vi "_Main_LookOnly_V2.0_3el_5el.vi"() -> ()   [LabVIEW 2017]
uses:
  <vilib>/Instr/_visa.llb/VISA Configure Serial Port (Instr).vi
panel:
  in  "5electrodes":bool=TRUE
  out "Channel 4, V":dbl format="%#_5g"
  in  "DAC 1 LIMIT, V":dbl min=-50.0 max=50.0 format="%#_5g"
  in  "DAC 2, V":dbl min=-10.0 max=10.0 format="%#_5g"
  in  "DAC 1, V":dbl min=-50.0 max=50.0 format="%#_5g"
  out "DAC1volt, V":dbl
  out "Field LOG":cluster{dbl[], dbl[]}(graph)
  out "Bytes at Port":u32
  out "RecTry":i32
  out "Field, kV/cm":dbl
  out "VoltageRes, V":dbl
  out "PlotPoints":cluster{"Time":dbl[], "Voltage":dbl[]}(graph)={"Time"=[0.0, 0.00037111111108161925, 0.000510833333311085, 0.0006505555555405509, 0.0007766666666915019, 0.0009172222221968695, 0.0010569444444263353, 0.0011958333333152243, 0.0013350000000274223], "Voltage"=[5.89, 5.89, 5.89, 5.89, 5.89, 5.89, 5.89, 5.89, 5.89]}
  out "VoltageBelow, V":dbl
  out "Current, mA":dbl format="%#_4g"
  out "Channel 3, V":dbl format="%#_5g"
  out "Channel 2, V":dbl format="%#_5g"
  out "Channel 1, V":dbl format="%#_5g"
  in  "Stop Button":bool
  in  "Start Button":bool
  in  "film H, nm":dbl=50.0
  in  "COM port":refnum<visa-resource-name>
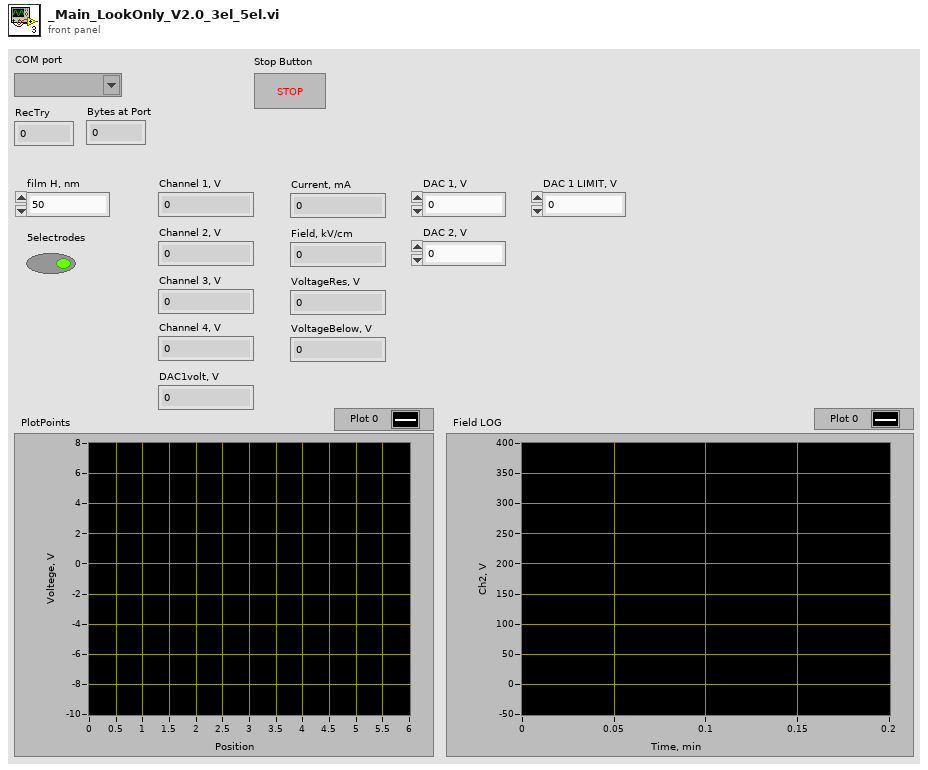
[diagram p1: front panel]
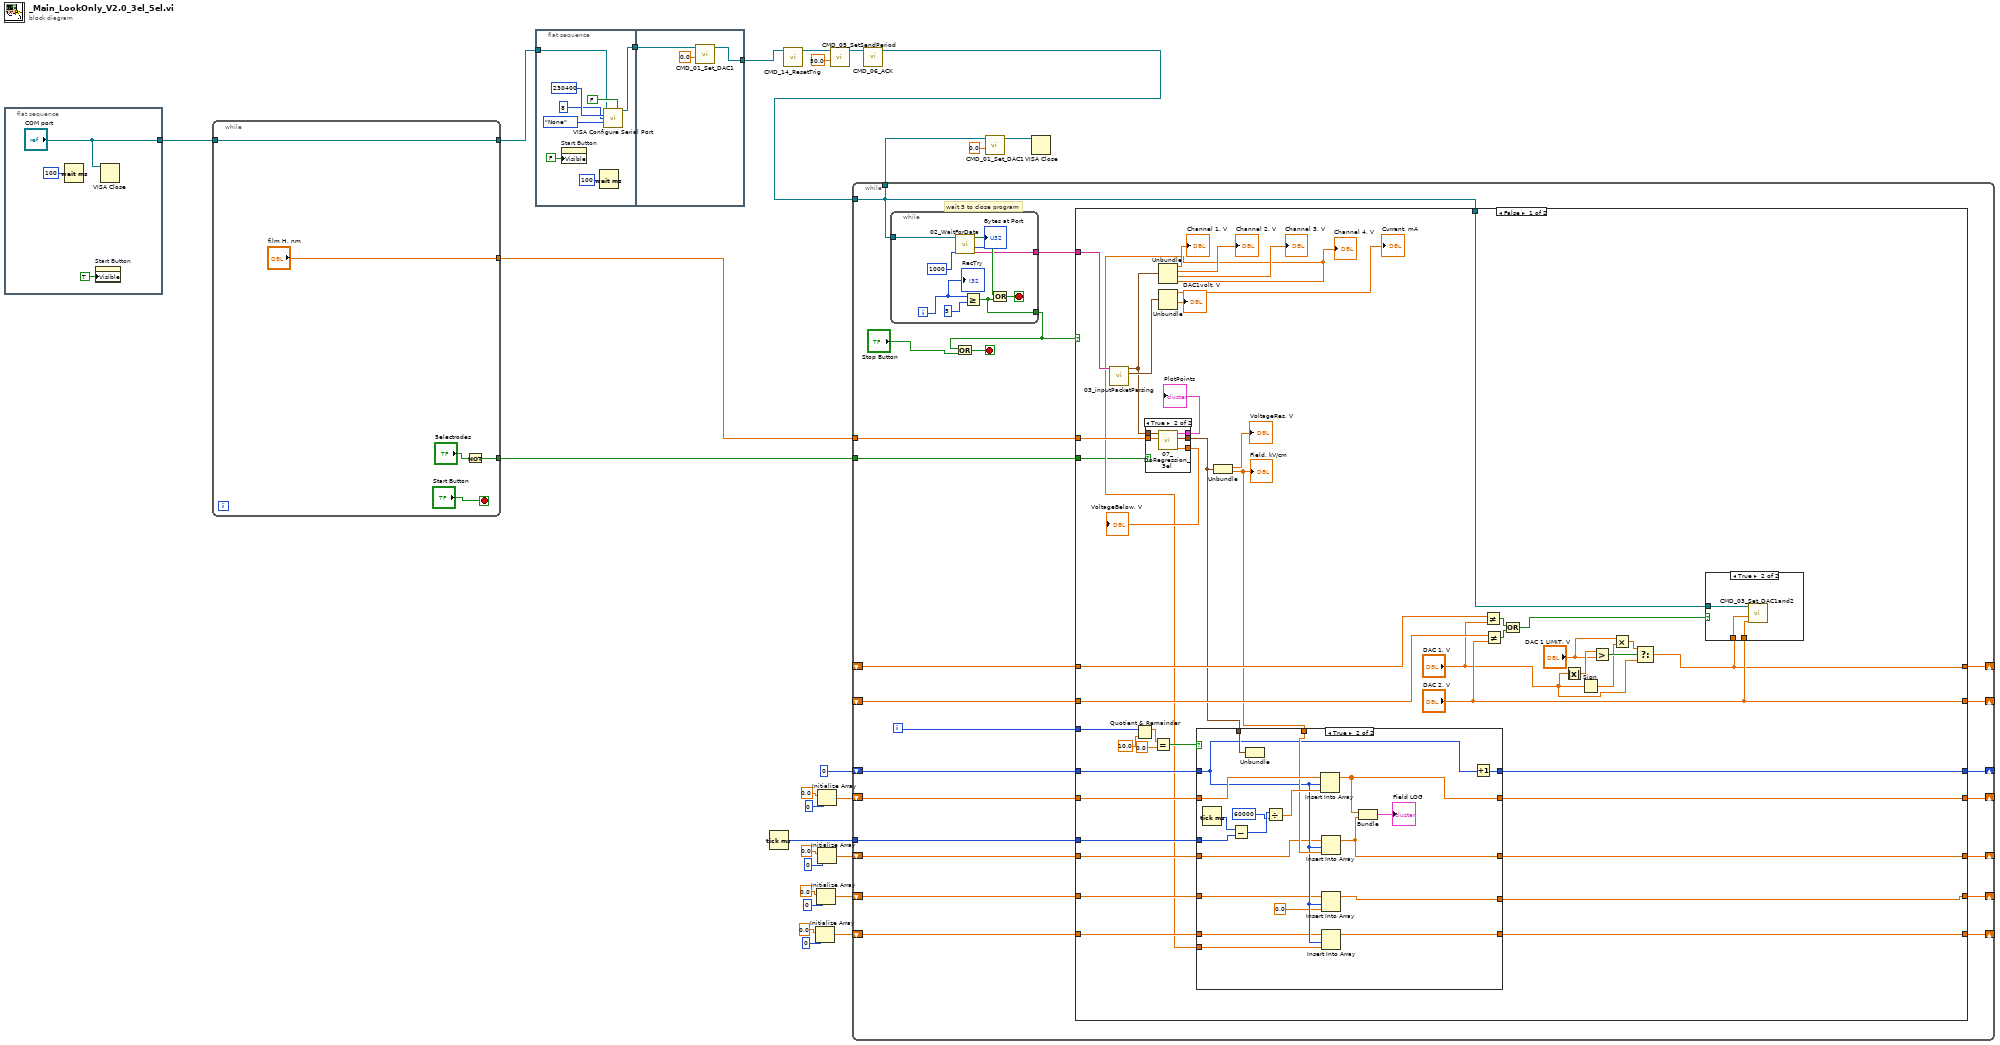
[diagram p0: block diagram]
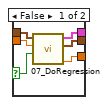
[diagram p2: hidden frame]
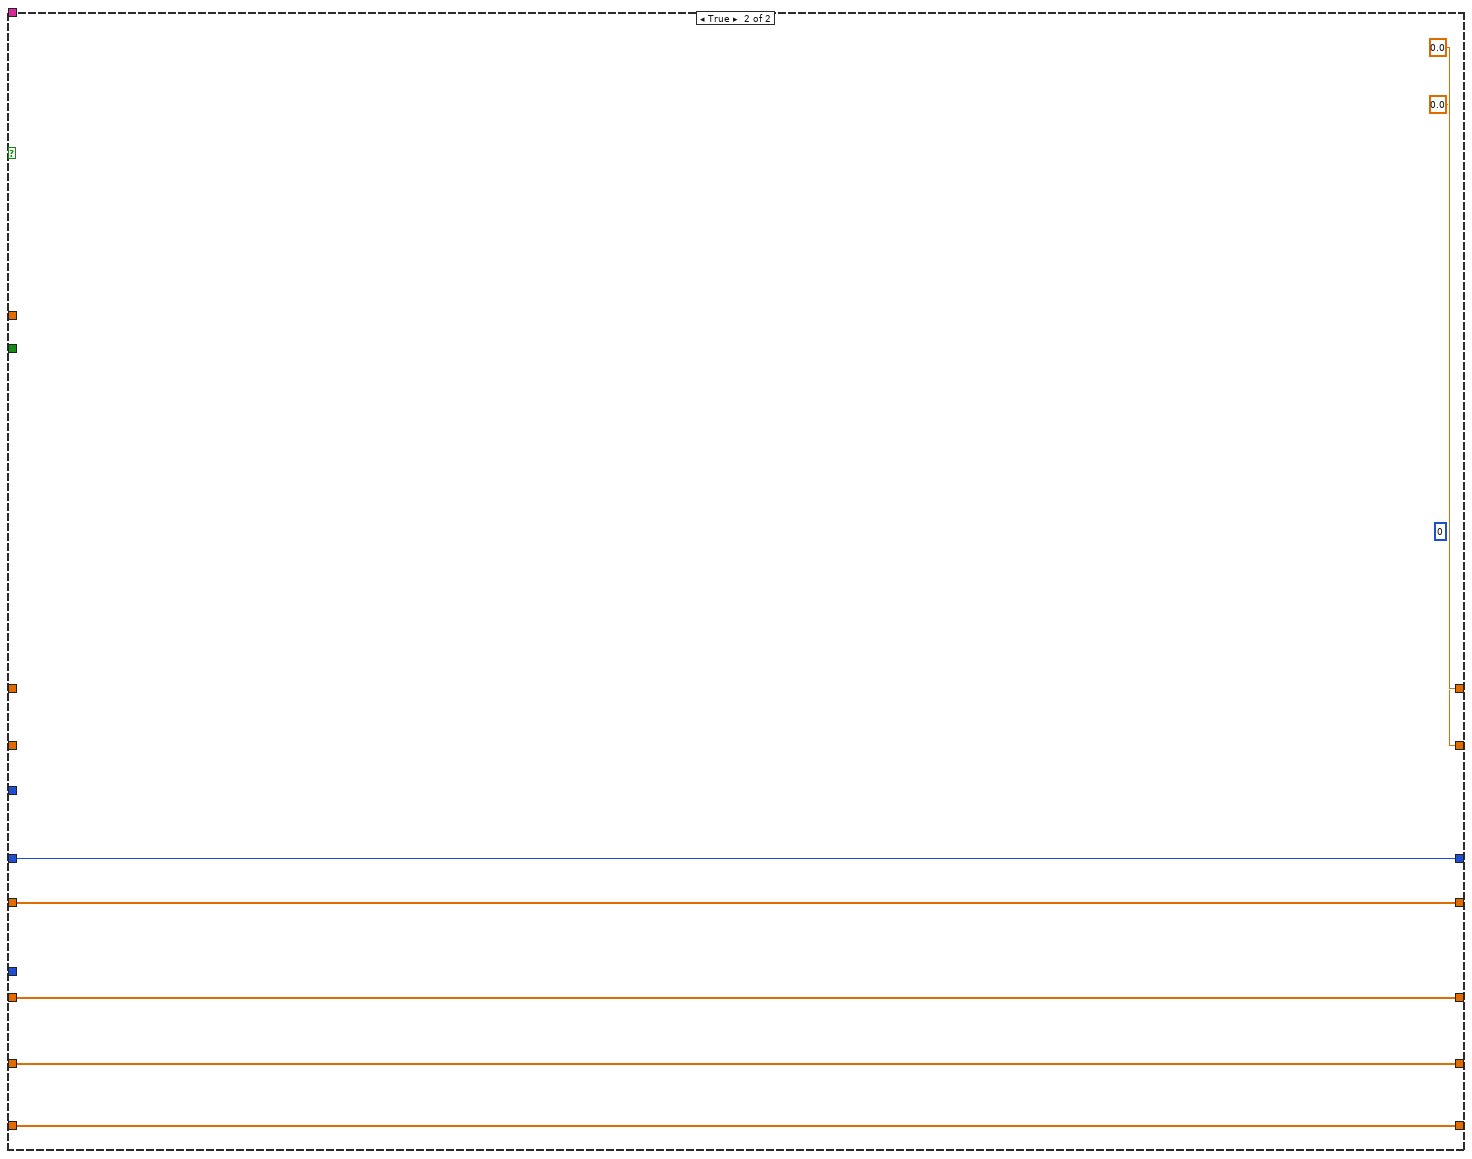
[diagram p5: hidden frame]
diagram:
  n1 = flat-sequence {
    tunnel: ["COM port"] -> w27
    frame #0 {
      n2 = Wait (ms)(milliseconds to wait=u32 100) -> ()  [unwired: 1 out]
      n3 = property on="Start Button" class="Bool"("Visible"=TRUE) -> ()  [unwired: 2 in, 2 out]
      n4 = VISA Close(VISA resource name="COM port") -> ()  [unwired: 1 in, 1 out]
    }
  }
  n5 = while {
    tunnel: w27 -> [w34]
    tunnel: [w34] -> w26
    tunnel: ["film H, nm"] -> w25
    tunnel: [w32] -> w1
    stop <- "Start Button" stop-if-true
    n6 = Not(x="5electrodes") -> (.not. x?=w32:bool)
  }
  n7 = flat-sequence {
    tunnel: w26 -> [w39]
    tunnel: [w38] -> w16
    tunnel: [w46] -> w23
    tunnel: w16 -> [w45]
    frame #0 {
      n8 = property on="Start Button" class="Bool"("Visible"=FALSE) -> ()  [unwired: 2 in, 2 out]
      n9 = Wait (ms)(milliseconds to wait=u32 100) -> ()  [unwired: 1 out]
      n10 = call-poly "VISA Configure Serial Port"("VISA resource name"=w39, "Enable Termination\nChar (T)"=FALSE ("Enable Termination\nChar (T)"), "baud rate (9600)"=u32 230400, "data bits (8)"=u16 8, "parity (0:none)"=enum16{"None", "Odd", "Even", "Mark", "Space"}."None") -> ("VISA resource name out"=w38:refnum<visa-resource-name>)  [unwired: 9 in, 1 out]
    }
    frame #1 {
      n11 = call "CMD_01_Set_DAC1.vi"("Input, V"=0.0, "VISA resource name"=w45) -> ("VISA resource name out"=w46:refnum<visa-resource-name>)  [unwired: 9 in]
    }
  }
  n12 = Tick Count (ms)() -> (millisecond timer value=w11:u32)
  n13 = call "CMD_14_ResetTrig.vi"("VISA resource name"=w23) -> ("VISA resource name out"=w19:refnum<visa-resource-name>)  [unwired: 10 in]
  n14 = Initialize Array(0.0 ("element"), 0 ("dimension size")) -> (w2:dbl[])
  n15 = Initialize Array(0.0 ("element"), 0 ("dimension size")) -> (w3:dbl[])
  n16 = Initialize Array(0.0 ("element"), 0 ("dimension size")) -> (w8:dbl[])
  n17 = Initialize Array(0.0 ("element"), 0 ("dimension size")) -> (w12:dbl[])
  n18 = call "CMD_05_SetSendPeriod.vi"("Period, ms"=50.0, "VISA resource name"=w19) -> ("VISA resource name out"=w18:refnum<visa-resource-name>)  [unwired: 9 in]
  n19 = call "CMD_06_ACK.vi"("VISA resource name"=w18) -> ("VISA resource name out"=w17:refnum<visa-resource-name>)  [unwired: 10 in]
  n20 = while {
    tunnel: w17 -> [w64]
    tunnel: [w64] -> w24
    tunnel: w25 -> [w66]
    shift-right: [w62] -> _
    shift-left: 0 -> [w63]
    tunnel: w11 -> [w60]
    shift-right: [w58] -> _
    shift-left: w12 -> [w61]
    shift-right: [w57] -> _
    shift-left: w8 -> [w59]
    shift-right: [w55] -> _
    shift-left: _ -> [w52]
    shift-right: [w54] -> _
    shift-left: _ -> [w53]
    shift-right: [w49] -> _
    shift-left: w3 -> [w51]
    shift-right: [w48] -> _
    shift-left: w2 -> [w50]
    tunnel: w1 -> [w47]
    i -> [w65]
    stop <- w69 stop-if-true
    # "wait 5 to close program"
    n21 = while {
      tunnel: w64 -> [w162]
      tunnel: [w165] -> w68
      tunnel: [w166] -> w67
      i -> [w164]
      stop <- w168 stop-if-true
      n22 = call "02_WaitForData.vi"("WaitTimeoutMS"=u32 1000, "VISA"=w162) -> ("Buffer"=w166:string, "Bytes at Port"=→"Bytes at Port":u32, "Data Recived"=w167:bool)  [unwired: 7 in]
      n23 = Greater Or Equal?(x=w164, y=5) -> (x >= y?=w165:bool)
      n24 = Or(x=w167, y=w165) -> (x .or. y?=w168:bool)
      "RecTry" <- w164
    }
    n25 = Or(x=w68, y="Stop Button") -> (x .or. y?=w69:bool)
    n26 = case shown="False" w68 {
      tunnel: w67 -> [w115 _]
      tunnel: w66 -> [w81 _]
      tunnel: w65 -> [w108 _]
      tunnel: w64 -> [w91 _]
      tunnel: w63 -> [w106 w161]
      tunnel: [w105 w161] -> w62
      tunnel: w61 -> [w104 w160]
      tunnel: w60 -> [w103 _]
      tunnel: w59 -> [w102 w159]
      tunnel: [w100 w160] -> w58
      tunnel: [w99 w159] -> w57
      tunnel: [w85 0.0 ("DAC 1, V")] -> w55
      tunnel: ["DAC 2, V" 0.0 ("DAC 2, V")] -> w54
      tunnel: w53 -> [w95 _]
      tunnel: w52 -> [w94 _]
      tunnel: w51 -> [w77 w156]
      tunnel: w50 -> [w76 w155]
      tunnel: [w75 w156] -> w49
      tunnel: [w74 w155] -> w48
      tunnel: w47 -> [w70 _]
      frame False {
        n27 = call "03_inputPacketParsing.vi"("string"=w115) -> ("DAC state"=w113:cluster{dbl, dbl, dbl, dbl}, "Voltage"=w80:cluster{dbl, dbl, dbl, dbl})  [unwired: 6 in, 3 out]
        n28 = Quotient & Remainder(x=w108, y=10.0) -> (x-y*floor(x/y)=w111:dbl)  [unwired: 1 out]
        n29 = case shown="True" w70 {
          selector: w70 -> [w118 _]
          tunnel: [w121 w126] -> w82
          tunnel: w81 -> [w117 w125]
          tunnel: w80 -> [w116 w124]
          tunnel: [w120 w123] -> w79
          tunnel: [w119 w122] -> w78
          frame False {
            n30 = call "07_DoRegression.vi"("6 electrodes"=w118, "film H, nm"=w117, "Input ChVoltage"=w116) -> ("VoltageBelow, V"=w119:dbl, "Regression"=w120:cluster{"VoltageRes, V":dbl, "Field, kV/cm":dbl}, "PlotPoints"=w121:cluster{"Time":dbl[], "Voltage":dbl[]})  [unwired: 6 in]
          }
          frame True {
            n31 = call "07_DoRegression_3el.vi"("film H, nm"=w125, "Input ChVoltage"=w124) -> ("VoltageBelow, V"=w122:dbl, "Regression"=w123:cluster{"VoltageRes, V":dbl, "Field, kV/cm":dbl}, "PlotPoints"=w126:cluster{"Time":dbl[], "Voltage":dbl[]})  [unwired: 7 in]
          }
        }
        "VoltageBelow, V" <- w78
        "PlotPoints" <- w82
        n32 = Equal?(x=w111, y=0.0) -> (x = y?=w107:bool)
        n33 = Unbundle(w80) -> (→"Channel 1, V":dbl, →"Channel 2, V":dbl, →"Channel 3, V":dbl, w71:dbl)
        "Channel 4, V" <- w71
        n34 = Unbundle(w113) -> (→"Current, mA":dbl, →"DAC1volt, V":dbl)  [unwired: 2 out]
        n35 = Unbundle(w79) -> ("VoltageRes, V"=→"VoltageRes, V":dbl, "Field, kV/cm"=w83:dbl)
        "Field, kV/cm" <- w83
        n36 = case shown="True" w107 {
          tunnel: w106 -> [w134 w144]
          tunnel: [w134 w149] -> w105
          tunnel: w79 -> [_ w154]
          tunnel: w104 -> [w132 w147]
          tunnel: w103 -> [_ w152]
          tunnel: w102 -> [w133 w143]
          tunnel: [w133 w139] -> w99
          tunnel: [w132 w146] -> w100
          tunnel: w83 -> [_ w145]
          tunnel: w77 -> [w131 w142]
          tunnel: w76 -> [w130 w141]
          tunnel: [w131 w137] -> w75
          tunnel: [w130 w138] -> w74
          tunnel: w71 -> [_ w140]
          frame False {
          }
          frame True {
            n37 = Tick Count (ms)() -> (millisecond timer value=w153:u32)
            n38 = Subtract(x=w153, y=w152) -> (x-y=w151:u32)
            n39 = Unbundle(w154) -> ()  [unwired: 2 out]
            n40 = Divide(x=w151, y=u32 60000) -> (x/y=w148:dbl)
            n41 = Insert Into Array(array=w147, index=w144, new element=w148) -> (w146:dbl[])
            n42 = Insert Into Array(array=w143, index=w144, new element=w145) -> (w139:dbl[])
            n43 = Insert Into Array(array=w142, index=w144, new element=0.0 ("new element/subarray")) -> (w137:dbl[])
            n44 = Insert Into Array(array=w141, index=w144, new element=w140) -> (w138:dbl[])
            n45 = Bundle(w146, w139) -> (→"Field LOG":cluster{dbl[], dbl[]})  [unwired: 1 in]
            n46 = Increment(x=w144) -> (x+1=w149:i32)
          }
        }
        n47 = Not Equal?(x=w94, y="DAC 1, V") -> (x != y?=w97:bool)
        n48 = Not Equal?(x=w95, y="DAC 2, V") -> (x != y?=w96:bool)
        n49 = Or(x=w97, y=w96) -> (x .or. y?=w93:bool)
        n50 = Absolute Value(x="DAC 1, V") -> (abs(x)=w90:dbl)
        n51 = Sign(1:"DAC 1, V") -> (0:w87:dbl)
        n52 = Greater?(x=w90, y="DAC 1 LIMIT, V") -> (0:w89:bool)
        n53 = Multiply(x="DAC 1 LIMIT, V", y=w87) -> (x*y=w88:dbl)
        n54 = Select(t=w88, s=w89, f="DAC 1, V") -> (s? t:f=w85:dbl)
        n55 = case shown="True" w93 {
          tunnel: "DAC 2, V" -> [_ w129]
          tunnel: w85 -> [_ w128]
          tunnel: w91 -> [_ w127]
          frame False {
          }
          frame True {
            n56 = call "CMD_03_Set_DAC1and2.vi"("Input2, V"=w129, "Input1, V"=w128, "VISA resource name"=w127) -> ()  [unwired: 8 in, 1 out]
          }
        }
      }
      frame True {
        (unwired) u32 0
      }
    }
  }
  n57 = call "CMD_01_Set_DAC1.vi"("Input, V"=0.0, "VISA resource name"=w24) -> ("VISA resource name out"=w21:refnum<visa-resource-name>)  [unwired: 9 in]
  n58 = VISA Close(VISA resource name=w21) -> ()  [unwired: 1 in, 1 out]
